vi "Increment Progress.vi"(11 "LUnit Test Suite in":refnum<class "LUnit Test Suite.lvclass">) -> (2 "Progress (%)":dbl, 3 "LUnit Test Suite out":refnum<class "LUnit Test Suite.lvclass">)   [LabVIEW 2020, in "LUnit Test Suite.lvclass"]
uses:
  LUnit Test Suite.lvclass
  LUnit Test Suite.lvclass/LUnit Test Suite.ctl
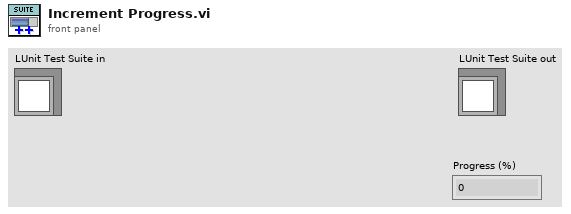
[diagram p1: front panel]
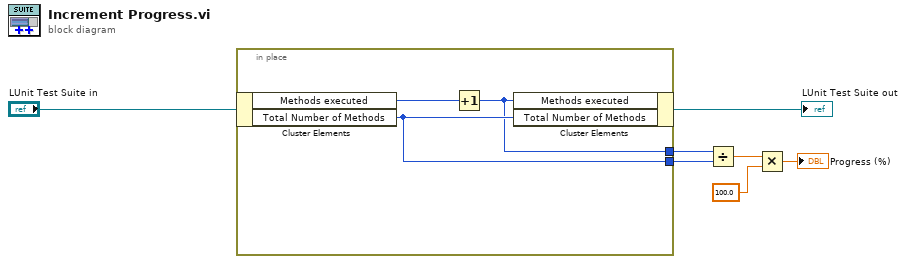
[diagram p0: block diagram]
diagram:
  n1 = in-place {
    in-place-border: [w9] -> w7
    in-place-border: [w8] -> w6
    n2 = in-place-cluster #1("LUnit Test Suite in") -> ("Methods executed"=w10:i32, "Total Number of Methods"=w9:i32)
    n3 = Increment(x=w10) -> (x+1=w8:i32)
    n4 = in-place-cluster #1("Methods executed"=w8, "Total Number of Methods"=w9) -> (→"LUnit Test Suite out":refnum<class "LUnit Test Suite.lvclass">)
  }
  n5 = Divide(x=w6, y=w7) -> (x/y=w5:dbl)
  n6 = Multiply(x=w5, y=100.0) -> (x*y=→"Progress (%)":dbl)
